vi "Test.vi"() -> ()   [LabVIEW 2017]
panel:
  in  "sigma":dbl
  in  "mu":dbl
  out "Histogram":dynamicdata(graph)
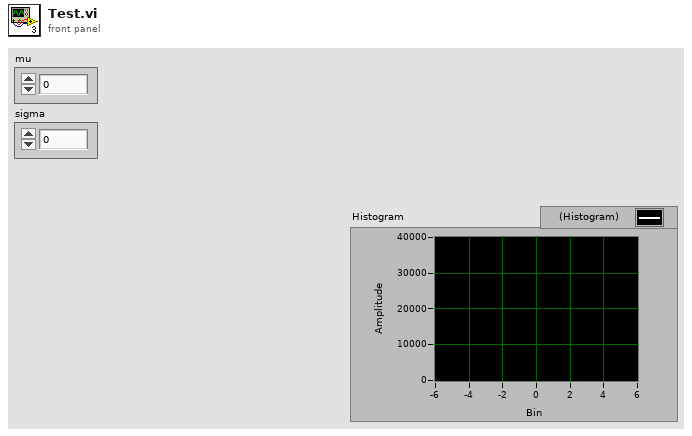
[diagram p1: front panel]
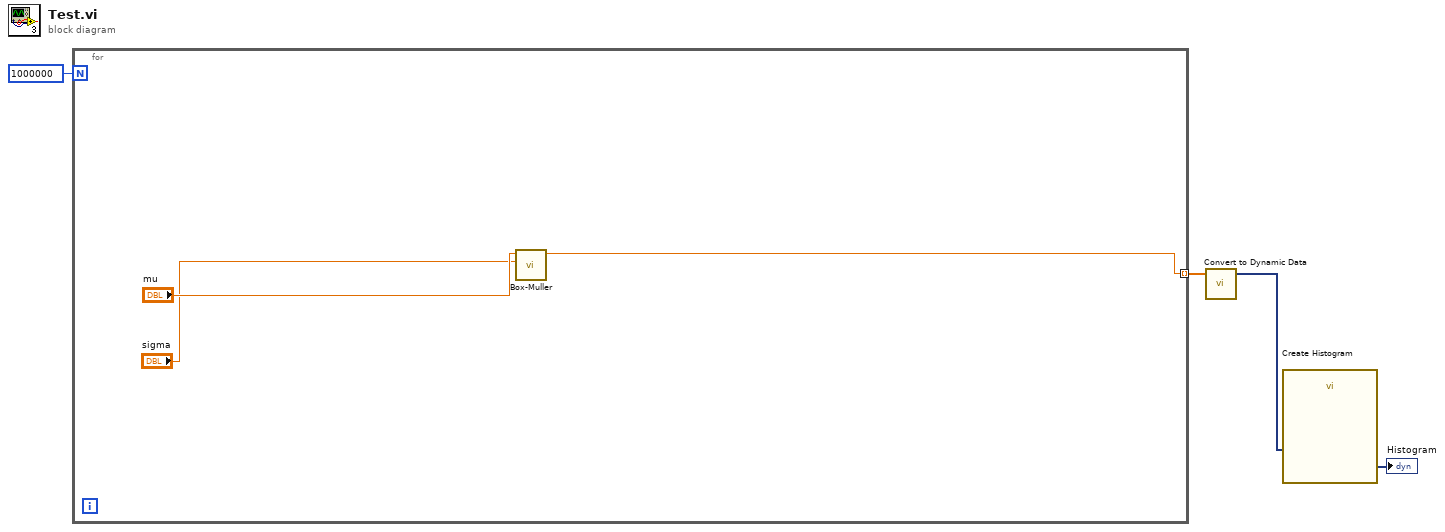
[diagram p0: block diagram]
diagram:
  n1 = for {
    N: 1000000 -> [_]
    tunnel: [w7] -> w1 mode=indexing
    n2 = call "Box-Muller.vi"("sigma"="sigma", "mu"="mu") -> ("Numeric Control"=w7:dbl)  [unwired: 9 in]
  }
  n3 = call "Convert to Dynamic Data"("Array"=w1) -> ("Dynamic Data Type"=w4:dynamicdata)  [unwired: 3 in]
  n4 = call "Create Histogram"("Signal"=w4) -> ("Histogram"=→"Histogram":dynamicdata)  [unwired: 9 in, 1 out]
